vi "UI_Log_In.vi"() -> ()   [LabVIEW 2014]
panel:
  in  "登录":bool
  in  "取消":bool
  in  "身份":u16(ring) items=["管理员", "普通用户"]
  in  "密码":string="123"
  in  "用户名":string="管理员1"
  # "欢迎使用\n\n                           轴承测试系统"
  # "版本:1.0\n\n\n  (c) 2015                  版权所有 *****************"
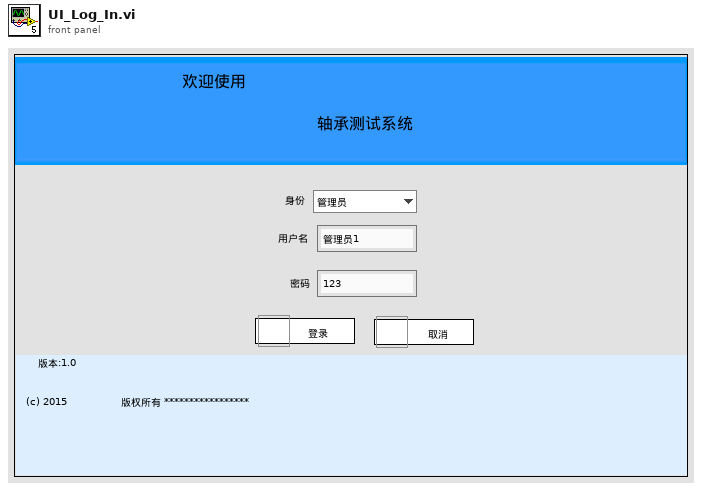
[diagram p1: front panel]
types:
  T1 = enum32{"Invalid", "Standard", "Closed", "Hidden", "Minimized", "Maximized"}
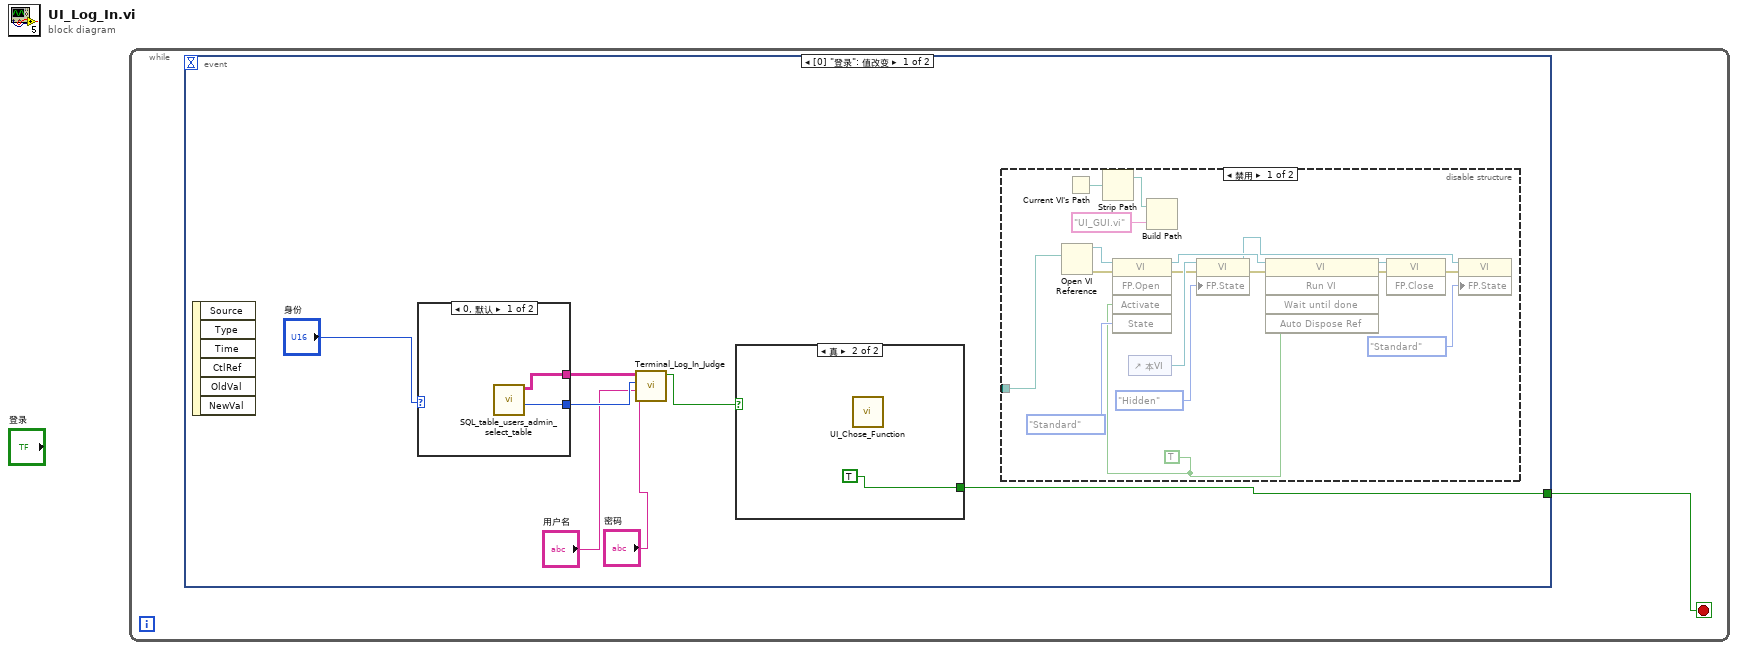
[diagram p0: block diagram]
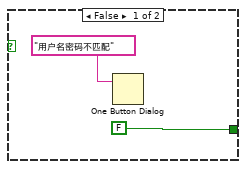
[diagram p3: hidden frame]
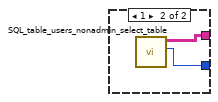
[diagram p4: hidden frame]
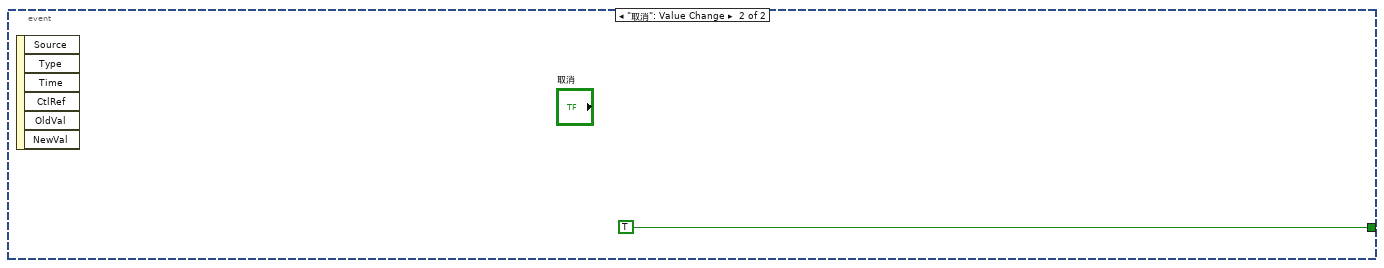
[diagram p5: hidden frame]
diagram:
  n1 = while {
    stop <- w1 stop-if-true
    n2 = event shown="[0] \"登录\": 值改变" {
      selector: _ -> [_ _]
      dyn-events: _ -> [_ _]
      timeout: _ -> [_ _]
      tunnel: [w2 TRUE] -> w1
      event "登录": Value Change {
        n3 = event-data() -> ()  [unwired: 1 in, 6 out]
        n4 = case shown="0, 默认" "身份" {
          tunnel: [w32 w34] -> w7
          tunnel: [w31 w33] -> w6
          frame 0, Default {
            n5 = call "SQL_table_users_admin_select_table.vi"() -> ("管理员个数"=w31:i32, "管理员信息"=w32:string[][])  [unwired: 9 in, 1 out]
          }
          frame 1 {
            n6 = call "SQL_table_users_nonadmin_select_table.vi"() -> ("普通用户个数"=w33:i32, "普通用户信息"=w34:string[][])  [unwired: 9 in, 1 out]
          }
        }
        n7 = call "Terminal_Log_In_Judge.vi"("密码"="密码", "用户名"="用户名", "用户个数"=w6, "用户名密码信息"=w7) -> ("用户名密码匹配"=w3:bool)  [unwired: 7 in]
        n8 = case shown="真" w3 {
          tunnel: [FALSE TRUE] -> w2
          frame False {
            n9 = One Button Dialog(message="用户名密码不匹配") -> ()  [unwired: 1 in, 1 out]
          }
          frame True {
            n10 = call "UI_Chose_Function.vi"() -> ()  [unwired: 12 in]
          }
        }
        n11 = disable-structure shown="禁用" {
          disable-tunnel: _ -> [w13 _]
          frame Disabled {
            w14 = TRUE ("激活？")
            n12 = Open VI Reference(vi path=w13) -> (vi reference=w27:refnum<vi>, error out=w26:errorcluster)  [unwired: 5 in]
            n13 = Current VI's Path() -> (path=w11:path)
            n14 = Strip Path(path=w11) -> (stripped path=w10:path)  [unwired: 1 out]
            n15 = invoke class="VI" method="FP.Open"(reference=w27, error in=w26, "Activate"=w14, "State"=T1."Standard" ("状态")) -> (reference out=w18:refnum<vi>, error out=w21:errorcluster)  [unwired: 1 in, 3 out]
            n16 = control-ref of="本VI"() -> (w22:refnum<vi>)
            n17 = Build Path(base path=w10, name or relative path="UI_GUI.vi" ("名称或相对路径")) -> (appended path=w12:path)
            n18 = property class="VI"(reference=w22, error in=w21, "FP.State"=T1."Hidden" ("前面板窗口:状态")) -> (reference out=w17:refnum<vi>, error out=w19:errorcluster)
            n19 = invoke class="VI" method="Run VI"(reference=w18, error in=w19, "Wait until done"=w14, "Auto Dispose Ref"=w14) -> (reference out=w24:refnum<vi>, error out=w23:errorcluster)  [unwired: 1 in, 3 out]
            n20 = invoke class="VI" method="FP.Close"(reference=w24, error in=w23) -> (error out=w16:errorcluster)  [unwired: 1 in, 2 out]
            n21 = property class="VI"(reference=w17, error in=w16, "FP.State"=T1."Standard" ("前面板窗口:状态")) -> ()  [unwired: 2 out]
          }
          frame Enabled {
          }
        }
      }
      event "取消": Value Change {
        n22 = event-data() -> ()  [unwired: 1 in, 6 out]
      }
    }
  }
